vi "VNA_Easy_Loop_Power Dependence.vi"(4 "Power Start (dbm)":dbl=-70.0, 5 "Transport":refnum<class "Transport.lvclass">, 6 "stop/span":dbl=700000000.0 format="%.2p", 7 "VNA Address":refnum<visa-resource-name>="GPIB0::15::INSTR", 8 "start/center":dbl=400000000.0 format="%.2p", 9 "sweep type (0 : linear)":u16(ring) items=["linear sweep", "logarithmic sweep", "frequency list", "CW time sweep", "power sweep"], 10 "sweep time (sec)":dbl=0.5 format="%.2f", 11 "num points":u16(ring)=8 items=["3", "11", "21 ('20) / 26 ('53)", "51", "101", "201", "401", "801", "1601"]) -> (2 "Polar plot":cluster{dbl[], sgl[]}[](graph))   [LabVIEW 2019]
uses:
  <instrlib>/Agilent 87XX Series/Agilent 87XX Series.lvlib
  <userlib>/LevyLab/Transport/Control Experiment/Control Experiment.lvclass
  <userlib>/LevyLab/Transport/Transport/Transport.lvclass
  <userlib>/LevyLab/Instrument Framework/Instrument Types/Cryostat/Instrument.Cryostat.lvclass
panel:
  in  "IF bandwidth":u16(ring)=3 items=["10 HZ", "30 HZ", "100 HZ", "300 HZ", "1000 HZ", "3000 HZ"]
  in  "Power Step (dbm)":dbl=0.1
  in  "Power End (dbm)":dbl=-5.0
  out "Data 2":cluster{dbl[], dbl[]}[](graph)
  out "B Field (T)":dbl
  out "Temperature (K)":dbl=0.018587874153063663
  in  "Vg (V)":dbl
  in  "Ids (mA)":dbl=9.55
  in  "Vds (V)":dbl=1.3
  in  "Experiment Description":string="B=0T\nT<30mK\nVbg(AO6) = 0V\nPower: -70 dbm to -5 dbm, 0.1 dbm step\nVd: 1.3V\nId: 9.55mA \nIFBW = 300 Hz \n400MHz to 700MHz"
  in  "Experiment Folder":string="03-Powersweep"
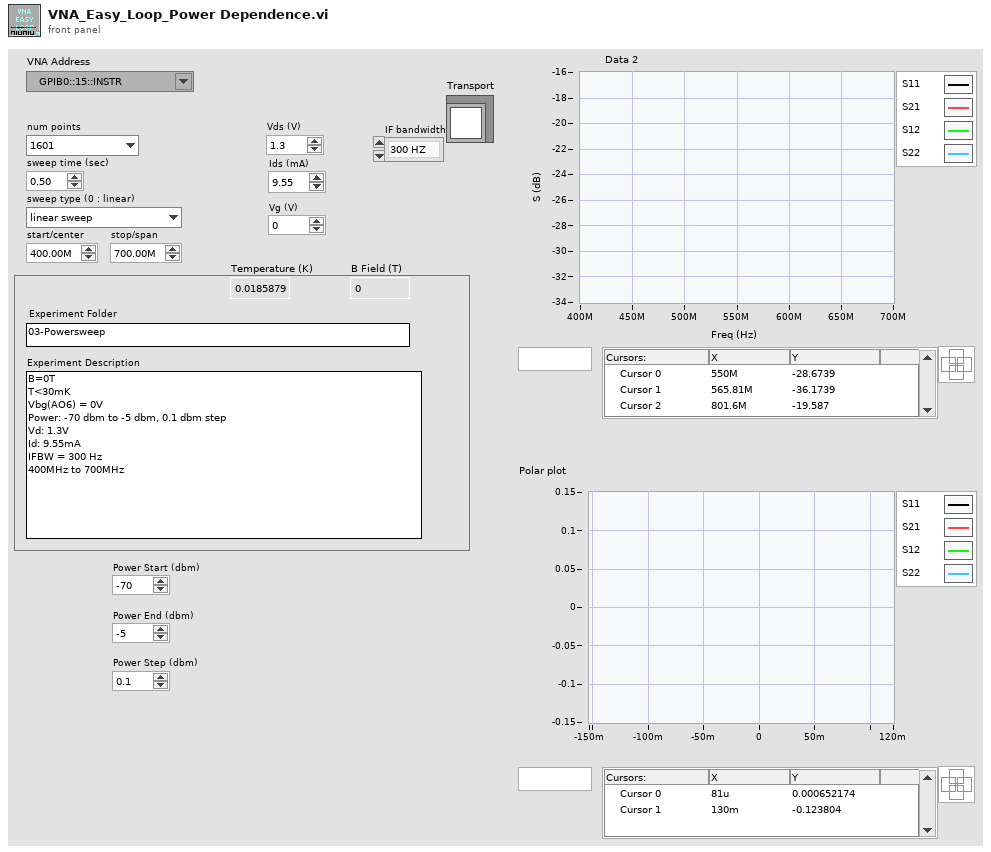
[diagram p1: front panel]
types:
  T1 = enum32{"Bad", "Idle", "Run top level", "Running"}
  T2 = typedef "Control Experiment.lvclass/Instrument Classes--cluster.ctl" = cluster{"DAQ":refnum<class "Instrument.LockinAPI.lvclass">, "Amplifier":refnum<class "Instrument.Amplifier.lvclass">, "Temperature":refnum<class "Instrument.Cryostat.lvclass">, "Magnet":refnum<class "Instrument.Cryostat.lvclass">, "Rotator":refnum<class "Instrument.Cryostat.lvclass">, "Level":refnum<class "Instrument.Cryostat.lvclass">, "Capacitance":refnum<class "Instrument.CBridge.lvclass">, "Delay Line":refnum<class "Instrument.DelayLine.lvclass">, "Strain Cell":refnum<class "Instrument.Strain.lvclass">, "VNA":refnum<class "Instrument.VNA.lvclass">, "Source":refnum<class "Instrument.VSource.lvclass">}
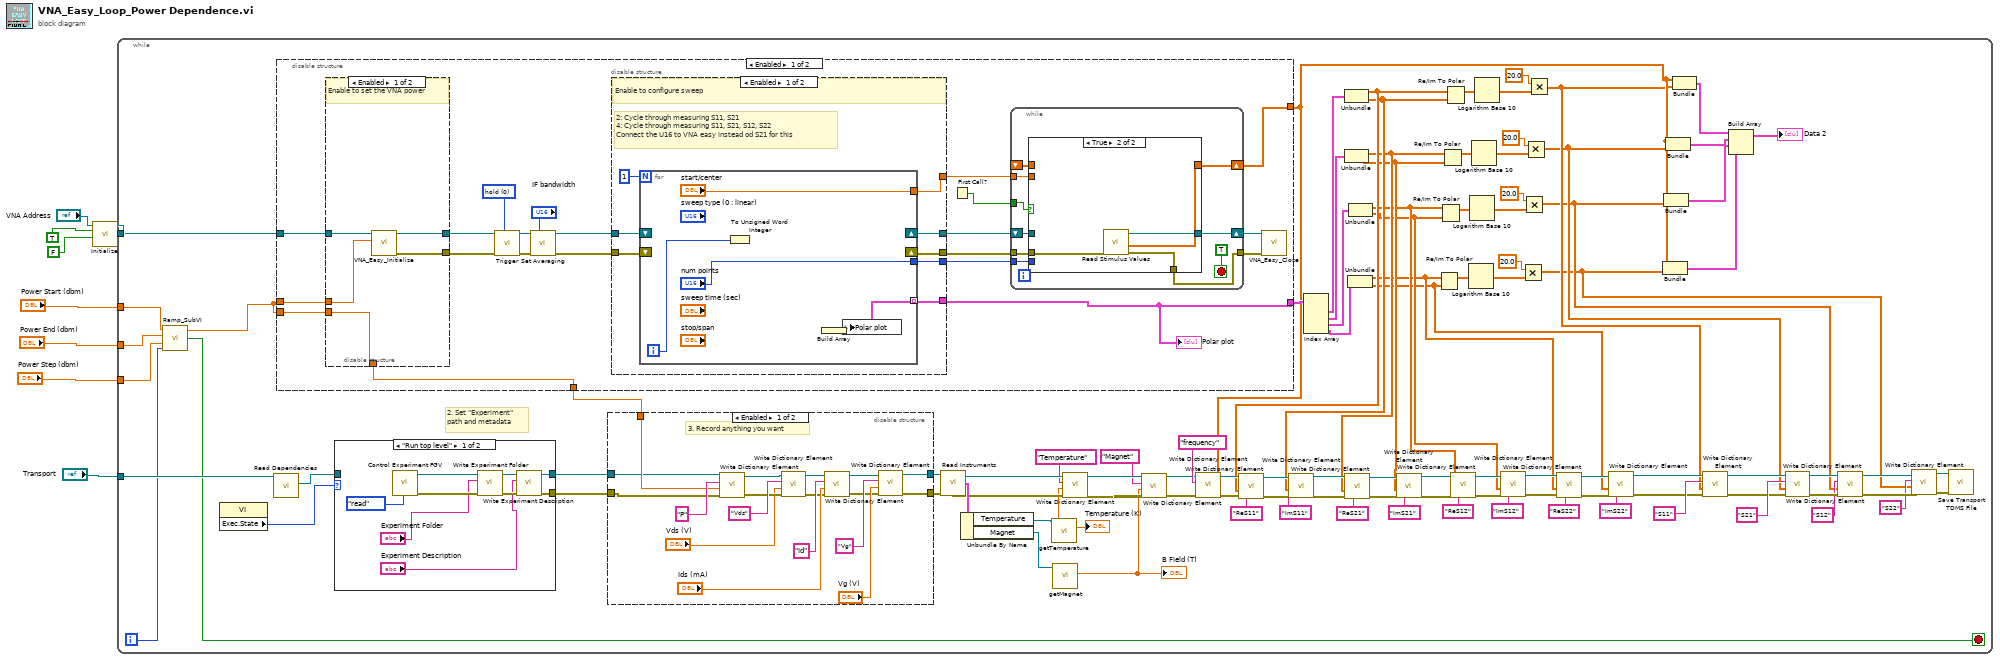
[diagram p0: block diagram]
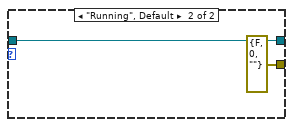
[diagram p2: hidden frame]
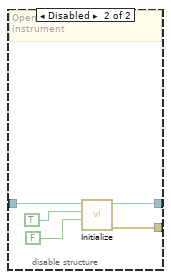
[diagram p5: hidden frame]
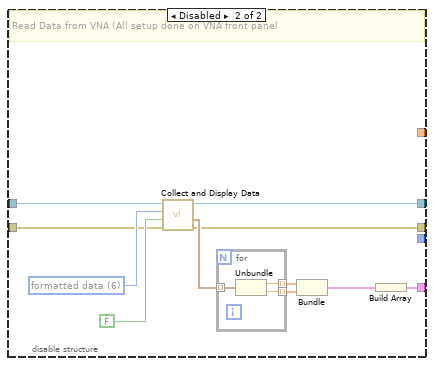
[diagram p6: hidden frame]
diagram:
  n1 = call <instrlib>:"Initialize.vi"("reset"=FALSE, "ID query"=TRUE, "VISA resource name"="VNA Address") -> ("VISA resource name out"=w3:refnum<visa-resource-name>)  [unwired: 7 in, 1 out]
  n2 = while {
    tunnel: "Transport" -> [w74]
    tunnel: "Power Start (dbm)" -> [w14]
    tunnel: w3 -> [w15]
    tunnel: "Power End (dbm)" -> [w13]
    tunnel: "Power Step (dbm)" -> [w12]
    i -> [w11]
    stop <- w10 stop-if-true
    # "2. Set \"Experiment\"\npath and metadata"
    n3 = call <userlib>:"Ramp_SubVI.vi"("index"=w11, "step"=w12, "end"=w13, "start"=w14) -> ("Stop?"=w10:bool, "Numeric"=w9:dbl)  [unwired: 1 in]
    n4 = property class="VI"() -> ("Exec.State"=w77:T1)  [unwired: 2 in, 2 out]
    n5 = call <userlib>:"Read Dependencies.vi"("Transport"=w74) -> ("C.E."=w73:refnum<class "Control Experiment.lvclass">)  [unwired: 8 in, 2 out]
    n6 = disable-structure shown="Enabled" {
      disable-tunnel: [w153 _] -> w72
      disable-tunnel: [w159 _] -> w103
      disable-tunnel: [w160 _] -> w30
      disable-tunnel: w9 -> [w152 _]
      disable-tunnel: w9 -> [w151 _]
      disable-tunnel: w15 -> [w150 _]
      frame Enabled {
        w148 = u16 0 items=["hold", "single", "number of groups", "continuous"] ("trigger (1 : single)")
        n7 = disable-structure shown="Enabled" {
          disable-tunnel: w150 -> [w184 w187]
          disable-tunnel: [w183 w185] -> w143
          disable-tunnel: [w182 w186] -> w145
          disable-tunnel: [w181 _] -> w159
          disable-tunnel: w152 -> [w181 _]
          disable-tunnel: w151 -> [w180 _]
          frame Enabled {
            # "Enable to set the VNA power"
            n8 = call "VNA_Easy_Initialize.vi"("Power (dbm)"=w180, "VISA Refnum in"=w184) -> ("error out"=w182:errorcluster, "VISA Refnum out"=w183:refnum<visa-resource-name>)  [unwired: 8 in]
          }
          frame Disabled {
            # "Open connection to instrument"
            n9 = call <instrlib>:"Initialize.vi"("reset"=FALSE, "ID query"=TRUE, "VISA resource name"=w187) -> ("error out"=w186:errorcluster, "VISA resource name out"=w185:refnum<visa-resource-name>)  [unwired: 7 in]
          }
        }
        n10 = call <instrlib>:"Trigger.vi"("trigger (1 : single)"=w148, "error in (no error)"=w145, "VISA resource name"=w143) -> ("error out"=w147:errorcluster, "VISA resource name out"=w146:refnum<visa-resource-name>)  [unwired: 7 in]
        n11 = call <instrlib>:"Set Averaging.vi"("VISA resource name"=w146, "IF bandwidth (5 : 3000 HZ)"="IF bandwidth", "error in (no error)"=w147) -> ("VISA resource name out"=w142:refnum<visa-resource-name>, "error out"=w144:errorcluster)  [unwired: 11 in]
        n12 = disable-structure shown="Enabled" {
          disable-tunnel: w142 -> [w197 w207]
          disable-tunnel: w144 -> [w196 w208]
          disable-tunnel: [w195 w205] -> w158
          disable-tunnel: [w194 w206] -> w162
          disable-tunnel: [w193 w203] -> w153
          disable-tunnel: [w191 _] -> w156
          disable-tunnel: [w190 _] -> w155
          frame Enabled {
            # "2: Cycle through measuring S11, S21\n4: Cycle through measuring S11, S21, S12, S22\nConnect the U16 to VNA easy instead od S21 for this"
            # "Enable to configure sweep"
            n13 = for {
              N: 1 -> [_]
              tunnel: [w198] -> w193 mode=indexing
              shift-right: [_] -> w194
              shift-left: w197 -> [_]
              shift-right: [_] -> w195
              shift-left: w196 -> [_]
              tunnel: ["start/center"] -> w191
              tunnel: ["num points"] -> w190
              i -> [w202]
              n14 = To Unsigned Word Integer(number=w202) -> ()  [unwired: 1 out]
              n15 = Build Array(w198) -> (w199:void[])
              n16 = local write "Polar plot"(w199) -> ()
            }
          }
          frame Disabled {
            w213 = u16 6 items=["raw data array 1", "raw data array 2", "raw data array 3", "raw data array 4", "error-corrected data", "error-corrected trace memory", "formatted data", "formatted memory", "formatted data / memory", "formatted data - memory"] ("data type (6 : formatted data)")
            # "Read Data from VNA (All setup done on VNA front panel"
            n17 = call <instrlib>:"Collect and Display Data.vi"("error in (no error)"=w208, "save to file"=FALSE, "data type (6 : formatted data)"=w213, "VISA resource name"=w207) -> ("error out"=w205:errorcluster, "data values"=w210:cluster{"real / stim":dbl, "imag / resp":sgl}[], "VISA resource name out"=w206:refnum<visa-resource-name>)  [unwired: 4 in, 1 out]
            n18 = for {
              tunnel: w210 -> [w216] mode=indexing
              tunnel: [w215] -> w211 mode=indexing
              tunnel: [w214] -> w212 mode=indexing
              n19 = Unbundle(w216) -> ("real / stim"=w215:dbl, "imag / resp"=w214:sgl)
            }
            n20 = Bundle(w211, w212) -> (w204:cluster{dbl[], sgl[]})  [unwired: 1 in]
            n21 = Build Array(w204) -> (w203:cluster{dbl[], sgl[]}[])
          }
        }
        "Polar plot" <- w153
        n22 = First Call?() -> (First Call?: T/F=w154:bool)
        n23 = while {
          shift-right: [w171] -> w161
          shift-left: w162 -> [w172]
          shift-right: [w169] -> w160
          shift-left: _ -> [w168]
          tunnel: w154 -> [w167]
          tunnel: w158 -> [w166]
          tunnel: [w165] -> w157
          tunnel: w156 -> [w164]
          tunnel: w155 -> [w163]
          stop <- TRUE stop-if-true
          n24 = case shown="True" w167 {
            tunnel: w172 -> [w174 _]
            tunnel: [w174 w179] -> w171
            tunnel: [w175 w176] -> w169
            tunnel: w168 -> [w175 _]
            tunnel: w166 -> [w173 w178]
            tunnel: [w173 w177] -> w165
            tunnel: w164 -> [_ _]
            tunnel: w163 -> [_ _]
            frame False {
            }
            frame True {
              n25 = call <instrlib>:"Read Stimulus Values.vi"("error in (no error)"=w178) -> ("error out"=w177:errorcluster, "stimulus list"=w176:dbl[], "VISA resource name out"=w179:refnum<visa-resource-name>)  [unwired: 8 in]
            }
          }
        }
        n26 = call "VNA_Easy_Close.vi"("error in (no error)"=w157, "VISA Refnum in"=w161) -> ()  [unwired: 9 in, 1 out]
      }
      frame Disabled {
      }
    }
    n27 = case shown="\"Run top level\"" w77 {
      tunnel: [w115 errorcluster {"status"=FALSE, "code"=0, "source"=""} ("error out")] -> w75
      tunnel: [w114 w121] -> w76
      tunnel: w73 -> [_ w121]
      frame "Run top level" {
        n28 = call <userlib>:"Control Experiment FGV.vi"("Function"=enum16{"read", "write"}."read") -> ("error out"=w118:errorcluster, "Control Experiment.lvclass out"=w119:refnum<class "Control Experiment.lvclass">)  [unwired: 9 in]
        n29 = call <userlib>:"Write Experiment Folder.vi"("error in (no error)"=w118, "Experiment Folder"="Experiment Folder", "Control Experiment in"=w119) -> ("error out"=w116:errorcluster, "Control Experiment out"=w117:refnum<class "Control Experiment.lvclass">)  [unwired: 7 in]
        n30 = call <userlib>:"Write Experiment Description.vi"("error in (no error)"=w116, "Experiment Description"="Experiment Description", "Control Experiment in"=w117) -> ("error out"=w115:errorcluster, "Control Experiment out"=w114:refnum<class "Control Experiment.lvclass">)  [unwired: 7 in]
      }
      frame "Running", Default {
      }
    }
    n31 = disable-structure shown="Enabled" {
      disable-tunnel: w76 -> [w131 w141]
      disable-tunnel: w75 -> [w130 w140]
      disable-tunnel: [w136 w141] -> w102
      disable-tunnel: [w122 w140] -> w101
      disable-tunnel: w103 -> [w132 _]
      frame Enabled {
        # "3. Record anything you want"
        n32 = call <userlib>:"Write Dictionary Element.vi"("error in (no error)"=w130, "value"=w132, "key"="P", "Control Experiment in"=w131) -> ("error out"=w128:errorcluster, "Control Experiment out"=w129:refnum<class "Control Experiment.lvclass">)  [unwired: 6 in]
        n33 = call <userlib>:"Write Dictionary Element.vi"("error in (no error)"=w128, "value"="Vds (V)", "key"="Vds", "Control Experiment in"=w129) -> ("error out"=w125:errorcluster, "Control Experiment out"=w138:refnum<class "Control Experiment.lvclass">)  [unwired: 6 in]
        n34 = call <userlib>:"Write Dictionary Element.vi"("error in (no error)"=w125, "value"="Ids (mA)", "key"="Id", "Control Experiment in"=w138) -> ("error out"=w123:errorcluster, "Control Experiment out"=w137:refnum<class "Control Experiment.lvclass">)  [unwired: 6 in]
        n35 = call <userlib>:"Write Dictionary Element.vi"("error in (no error)"=w123, "value"="Vg (V)", "key"="Vg", "Control Experiment in"=w137) -> ("error out"=w122:errorcluster, "Control Experiment out"=w136:refnum<class "Control Experiment.lvclass">)  [unwired: 6 in]
      }
      frame Disabled {
      }
    }
    n36 = call <userlib>:"Read Instruments.vi"("error in (no error)"=w101, "Control Experiment in"=w102) -> ("error out"=w97:errorcluster, "Instruments"=w100:T2, "Control Experiment out"=w96:refnum<class "Control Experiment.lvclass">)  [unwired: 7 in]
    n37 = Unbundle By Name(w100) -> ("Temperature"=w98:refnum<class "Instrument.Cryostat.lvclass">, "Magnet"=w99:refnum<class "Instrument.Cryostat.lvclass">)
    n38 = call-dynamic "getTemperature.vi"("Instrument.Cryostat in"=w98) -> ("Temperature (K)"=w95:dbl)  [unwired: 6 in, 4 out]
    "Temperature (K)" <- w95
    n39 = call-dynamic "getMagnet.vi"("Instrument.Cryostat in"=w99) -> ("B Field (T)"=w88:dbl)  [unwired: 6 in, 4 out]
    "B Field (T)" <- w88
    n40 = call <userlib>:"Write Dictionary Element.vi"("error in (no error)"=w97, "value"=w95, "key"="Temperature", "Control Experiment in"=w96) -> ("error out"=w90:errorcluster, "Control Experiment out"=w93:refnum<class "Control Experiment.lvclass">)  [unwired: 6 in]
    n41 = call <userlib>:"Write Dictionary Element.vi"("error in (no error)"=w90, "value"=w88, "key"="Magnet", "Control Experiment in"=w93) -> ("error out"=w91:errorcluster, "Control Experiment out"=w92:refnum<class "Control Experiment.lvclass">)  [unwired: 6 in]
    n42 = call <userlib>:"Write Dictionary Element.vi"("error in (no error)"=w91, "value"=w30, "key"="frequency", "Control Experiment in"=w92) -> ("error out"=w62:errorcluster, "Control Experiment out"=w64:refnum<class "Control Experiment.lvclass">)  [unwired: 6 in]
    n43 = Index Array(array=w72) -> (element #1=w110:cluster{dbl[], sgl[]}, element #2=w104:cluster{dbl[], sgl[]}, element #3=w80:cluster{dbl[], sgl[]}, element #4=w78:cluster{dbl[], sgl[]})  [unwired: 4 in]
    n44 = Unbundle(w110) -> (w40:dbl[], w39:sgl[])
    n45 = call <userlib>:"Write Dictionary Element.vi"("error in (no error)"=w62, "value"=w40, "key"="ReS11", "Control Experiment in"=w64) -> ("error out"=w61:errorcluster, "Control Experiment out"=w63:refnum<class "Control Experiment.lvclass">)  [unwired: 6 in]
    n46 = call <userlib>:"Write Dictionary Element.vi"("error in (no error)"=w61, "value"=w39, "key"="ImS11", "Control Experiment in"=w63) -> ("error out"=w56:errorcluster, "Control Experiment out"=w58:refnum<class "Control Experiment.lvclass">)  [unwired: 6 in]
    n47 = Unbundle(w104) -> (w26:dbl[], w25:sgl[])
    n48 = call <userlib>:"Write Dictionary Element.vi"("error in (no error)"=w56, "value"=w26, "key"="ReS21", "Control Experiment in"=w58) -> ("error out"=w55:errorcluster, "Control Experiment out"=w57:refnum<class "Control Experiment.lvclass">)  [unwired: 6 in]
    n49 = Unbundle(w78) -> (w22:dbl[], w21:sgl[])
    n50 = Unbundle(w80) -> (w24:dbl[], w23:sgl[])
    n51 = call <userlib>:"Write Dictionary Element.vi"("error in (no error)"=w55, "value"=w25, "key"="ImS21", "Control Experiment in"=w57) -> ("error out"=w43:errorcluster, "Control Experiment out"=w44:refnum<class "Control Experiment.lvclass">)  [unwired: 6 in]
    n52 = Re/Im To Polar(2:w21, 3:w22) -> (1:w32:dbl[])  [unwired: 1 out]
    n53 = Re/Im To Polar(2:w23, 3:w24) -> (1:w35:dbl[])  [unwired: 1 out]
    n54 = Re/Im To Polar(2:w25, 3:w26) -> (1:w16:dbl[])  [unwired: 1 out]
    n55 = Re/Im To Polar(2:w39, 3:w40) -> (1:w68:dbl[])  [unwired: 1 out]
    n56 = call <userlib>:"Write Dictionary Element.vi"("error in (no error)"=w43, "value"=w24, "key"="ReS12", "Control Experiment in"=w44) -> ("error out"=w51:errorcluster, "Control Experiment out"=w52:refnum<class "Control Experiment.lvclass">)  [unwired: 6 in]
    n57 = Logarithm Base 10(1:w32) -> (0:w31:dbl[])
    n58 = Logarithm Base 10(1:w35) -> (0:w34:dbl[])
    n59 = Logarithm Base 10(1:w16) -> (0:w37:dbl[])
    n60 = Logarithm Base 10(1:w68) -> (0:w67:dbl[])
    n61 = call <userlib>:"Write Dictionary Element.vi"("error in (no error)"=w51, "value"=w23, "key"="ImS12", "Control Experiment in"=w52) -> ("error out"=w46:errorcluster, "Control Experiment out"=w48:refnum<class "Control Experiment.lvclass">)  [unwired: 6 in]
    n62 = Multiply(x=20.0, y=w31) -> (x*y=w17:dbl[])
    n63 = Multiply(x=20.0, y=w34) -> (x*y=w18:dbl[])
    n64 = Multiply(x=20.0, y=w37) -> (x*y=w19:dbl[])
    n65 = Multiply(x=20.0, y=w67) -> (x*y=w20:dbl[])
    n66 = call <userlib>:"Write Dictionary Element.vi"("error in (no error)"=w46, "value"=w22, "key"="ReS22", "Control Experiment in"=w48) -> ("error out"=w45:errorcluster, "Control Experiment out"=w47:refnum<class "Control Experiment.lvclass">)  [unwired: 6 in]
    n67 = call <userlib>:"Write Dictionary Element.vi"("error in (no error)"=w45, "value"=w21, "key"="ImS22", "Control Experiment in"=w47) -> ("error out"=w41:errorcluster, "Control Experiment out"=w42:refnum<class "Control Experiment.lvclass">)  [unwired: 6 in]
    n68 = Bundle("stimulus list"=w30, w17) -> (w27:cluster{"stimulus list":dbl[], dbl[]})  [unwired: 1 in]
    n69 = Bundle("stimulus list"=w30, w18) -> (w28:cluster{"stimulus list":dbl[], dbl[]})  [unwired: 1 in]
    n70 = Bundle("stimulus list"=w30, w19) -> (w29:cluster{"stimulus list":dbl[], dbl[]})  [unwired: 1 in]
    n71 = Bundle("stimulus list"=w30, w20) -> (w71:cluster{"stimulus list":dbl[], dbl[]})  [unwired: 1 in]
    n72 = call <userlib>:"Write Dictionary Element.vi"("error in (no error)"=w41, "value"=w20, "key"="S11", "Control Experiment in"=w42) -> ("error out"=w106:errorcluster, "Control Experiment out"=w105:refnum<class "Control Experiment.lvclass">)  [unwired: 6 in]
    n73 = Build Array(w71, w29, w28, w27) -> (→"Data 2":cluster{"stimulus list":dbl[], dbl[]}[])
    n74 = call <userlib>:"Write Dictionary Element.vi"("error in (no error)"=w106, "value"=w19, "key"="S21", "Control Experiment in"=w105) -> ("error out"=w84:errorcluster, "Control Experiment out"=w87:refnum<class "Control Experiment.lvclass">)  [unwired: 6 in]
    n75 = call <userlib>:"Write Dictionary Element.vi"("error in (no error)"=w84, "value"=w18, "key"="S12", "Control Experiment in"=w87) -> ("error out"=w83:errorcluster, "Control Experiment out"=w86:refnum<class "Control Experiment.lvclass">)  [unwired: 6 in]
    n76 = call <userlib>:"Write Dictionary Element.vi"("error in (no error)"=w83, "value"=w17, "key"="S22", "Control Experiment in"=w86) -> ("error out"=w79:errorcluster, "Control Experiment out"=w85:refnum<class "Control Experiment.lvclass">)  [unwired: 6 in]
    n77 = call <userlib>:"Save Transport TDMS File.vi"("error in (no error)"=w79, "Control Experiment in"=w85) -> ()  [unwired: 8 in, 2 out]
  }
